vi "AMC Send Local Message.vi"(4 "Message Attributes":T1, 6 "Priority Message (F)":bool, 7 "Process (\"\" - local)":string, 8 "error in (no error)":errorcluster, 9 "Message Value":string, 10 "Message Name":string, 11 "Message Queue in":T2) -> (0 "error out":errorcluster, 3 "Message Queue out":T2)   [LabVIEW 2013, in "main.lvlib" / "TLB_Dependencies.lvlib"]
doc: "This VI adds a message to the local message queue provided by the queue reference or to another message queue on the local target based on the receiver process name."
uses:
  TLB_Dependencies.lvlib
  amc_Message Queue.ctl
  amc_Message.ctl
  <vilib>/FTP/util/Keyed Array.ctl
  <vilib>/FTP/NI_FTP.lvlib
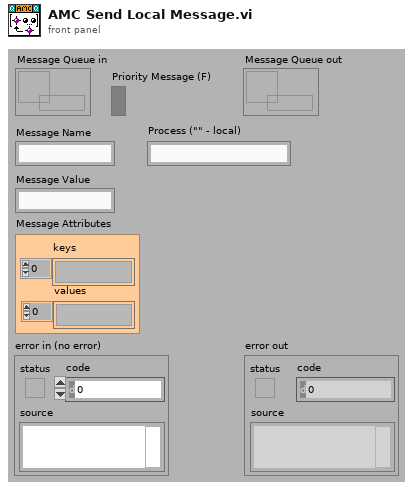
[diagram p1: front panel]
types:
  T1 = typedef "NI_FTP.lvlib/Keyed Array.ctl" = cluster{"keys":string[], "values":string[]}
  T2 = typedef "main.lvlib/TLB_Dependencies.lvlib/amc_Message Queue.ctl" = refnum<queue>
  T3 = typedef "main.lvlib/TLB_Dependencies.lvlib/amc_Message.ctl" = cluster{"Name":string, "Value":string, "Attributes":T1, "Receiver Host":string, "Receiver Process":string, "Source Host":string, "Source Process":string, "Priority Message":bool, "Acknowledge Message":bool}
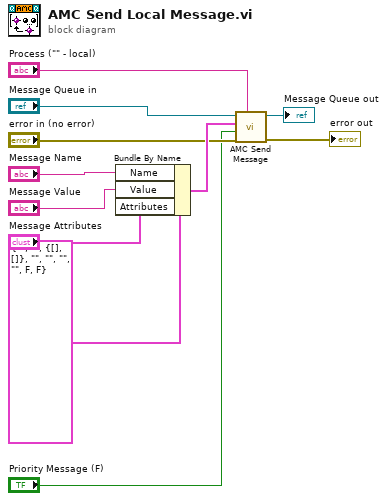
[diagram p0: block diagram]
diagram:
  n1 = Bundle By Name(cluster=T3 {"Name"="", "Value"="", "Attributes"={"keys"=[], "values"=[]}, "Receiver Host"="", "Receiver Process"="", "Source Host"="", "Source Process"="", "Priority Message"=FALSE, "Acknowledge Message"=FALSE} ("Message"), "Name"="Message Name", "Value"="Message Value", "Attributes"="Message Attributes") -> (w11:T3)
  n2 = call "AMC Send Message.vi"("Receiver Process"="Process (\"\" - local)", "error in (no error)"="error in (no error)", "Priority Message (F)"="Priority Message (F)", "Message"=w11, "Message Queue in"="Message Queue in") -> ("error out"=→"error out":errorcluster, "Message Queue out"=→"Message Queue out":T2)  [unwired: 3 in, 2 out]
